vi "Text control 2 v0.8.vi"() -> ()   [LabVIEW 2016]
panel:
  out "error out":errorcluster
  in  "Units":bool
  out "Elapsed Time":dbl caption="Elapsed Time (s)"
  out "Ion vs time":cluster{"Y data in":dbl[], "X data in":dbl[]}[](graph)
  out "Ig":dbl format="%.2e"
  out "Id":dbl format="%.2e"
  out "Is":dbl format="%.2e"
  out "I vs Vg":cluster{"Y data in":dbl[], "X data in":dbl[]}[](graph)
  in  "Panel Controls 2":T1={"Emergency Stop"=refnum, "TransGraph Max"=1e-05, "Text/Graph (text=false)"=TRUE, "TransGraph Min"=1e-11} {"TransGraph Min" format="%.2e"; "TransGraph Max" format="%.2e"}
  out "Currently running:":string="#output s 0 0 0 -0.008 0.008 0.002"
  in  "Lines left to run:":string
  in  "Standby":T2
  in  "Full Reset":bool
  in  "SMU4":cluster{"on/off":bool, "Voltage":dbl} {"Voltage" min=-100.0 max=100.0 format="%.2f"}
  in  "Source/Drain Range":u8(slide)=6 max=11 scale=0.0..11.0
  in  "Source/Drain\nRange mode":u16(ring) items=["Auto", "Limited", "Fixed"]
  in  "Gate Range":u8(slide)=6 max=11 scale=0.0..11.0
  in  "Gate Range\nmode":u16(ring) items=["Auto", "Limited", "Fixed"]
  in  "Gate":T3={"Gate Start"=0.0, "Gate Stop"=2.0, "Gate Step (linear only)"=1.0, "Gate Compliance"=0.0001, "Gate PComp"=0.0, "Range mode"=0, "Range"=6} {"Range" max=11 scale=0.0..11.0; "Range mode" items=["Auto", "Limited", "Fixed"]; "Gate PComp" format="%^.2e"; "Gate Compliance" format="%^.2e"; "Gate Step (linear only)" format="%^.4e"; "Gate Stop" format="%^.4e"; "Gate Start" format="%^.4e"}
  in  "Drain 2":T4={"Drain Start"=0.0, "Drain Stop"=2.0, "Drain Compliance"=0.0001, "Drain Step"=1.0, "Drain PComp"=0.0, "Range mode"=0, "Range"=6} {"Range" max=11 scale=0.0..11.0; "Range mode" items=["Auto", "Limited", "Fixed"]; "Drain PComp" format="%^.2e"; "Drain Step" format="%^.4e"; "Drain Compliance" format="%^.2e"; "Drain Stop" format="%^.4e"; "Drain Start" format="%^.4e"}
  in  "Timings 2":T5={"integration time"=0, "Short/Long integration time"=0.00064, "hold time (sec)"=0.0, "delay time (sec)"=0.0, "Step Time (0 disables)"=0.0, "sweep method"=0, "Pulse period"=0.005, "Base voltage"=0.0, "Pulse width"=0.0005} {"Pulse width" min=0.0005 max=0.1 step=0.0001 format="%.4f"; "Base voltage" format="%^.4e"; "Pulse period" min=0.005 max=1.0 step=0.0001 format="%.4f"; "sweep method" items=["Continuous", "Pulsed"]; "Step Time (0 disables)" format="%.2f"; "delay time (sec)" format="%.4f"; "hold time (sec)" format="%.4f"; "Short/Long integration time" format="%^.0e"; "integration time" scale=0.0..2.0}
  in  "Panel Controls":T6={"Emergency Stop"=refnum, "TransGraph Max"=1e-05, "Text/Graph (text=false)"=TRUE} {"TransGraph Max" format="%.2e"}
  in  "Interrupt run":bool
  in  "Drain: Compliance":dbl=0.001 format="%.8f"
  in  "Gate: Compliance":dbl=0.001 format="%.8f"
  out "Path":path=path "C:/users/rlp38/09Apr2009LTtesting/test2.txt"
  in  "hold time /s":dbl format="%.2f"
  in  "delay time /s":dbl format="%.2f"
  in  "integration time":u32(slide) max=2 step=1 scale=0.0..2.0
  in  "Integration time (short)":dbl=0.0019 min=8e-05 max=0.0019 step=8e-05 format="%^.0e"
  in  "Integration time (long)":dbl=0.32 min=0.04 max=2.0 step=0.02 format="%.2f"
  in  "Step delay /s":dbl format="%.2f"
  in  "Program":string="#pulsedstressV d 0.03 20 0 0.5 0.0827 5\n#\nitime s\ngaterangemode l\ndrainrangemode l\n#pulsed on 0.05 0 0.02\ntransfer d 1 -1 -0.1 -1 -1 0\nwait-min 1\ntransfer d 1 -1 -0.1 -1 -1 0\n#transfer d -10 40 1 5 40 35\n#transfer d -10 40 1 5 40 35\n#output d 0 40 20 0 40 1\n#\n#\n#sample 1 0.008 221 6 0.003\n#samplei 400e-6 200 6 0.002 0.1\n#vsu2pulse -10 4\n#\n#stressV 0.016 0.03 2e-4 0.1e-3 11\n#stressI 220e-7 0.08 15\n#transfer s -1 1 0.5 -0.005 0.005 0.005\n#output s 0 0 0 -0.008 0.008 0.002\n"
  # "Syntax:\nitime [s|m|l]\ngaterangemode [a|l|f]\ndrainrangemode [a|l|f]\npulsed [on|off] PulsePeriod(sec) PulseBaseVoltage PulseONWidth(sec)\nstandby [on l off]\nwait NumMilliseconds\nwait-min NumMinutes\n# texthere = comment\ntransfer [s|d] VgStart VgStop VgStep VdStart VdStop VdStep\noutput [s|d] VgStart VgStop VgStep VdStart VdStop VdStep\nsample Vg Vd NumSamples Time(s) SampleInterval(s)\nsamplei Idg NumSamples Time(s) SampleInterval(s) VDGcompliance\n# if in doubt use SampleInterval(s) = 0.004\nstressV VG VD IGcompliance IDcompliance Duration(sec)\nstressI IDG VDGcompliance Duration(sec)\nvsu2pulse Bias Duration(s)\npulsedstressV [s|d] VEstop VgON VgOFF Period(s) PulseONwidth(s) Vd\nsample-fpp Vg Vd NumSamples Time\nresample-fpp Vg Vd\ntransfer-fpp [s|d] VgStart VgStop VgStep VdStart VdStop VdStep\noutput-fpp [s|d] VgStart VgStop VgStep VdStart VdStop VdStep"
  # "Time"
  # "Sec"
  # "Min"
  # "100 samples is approx 13s with medium integration"
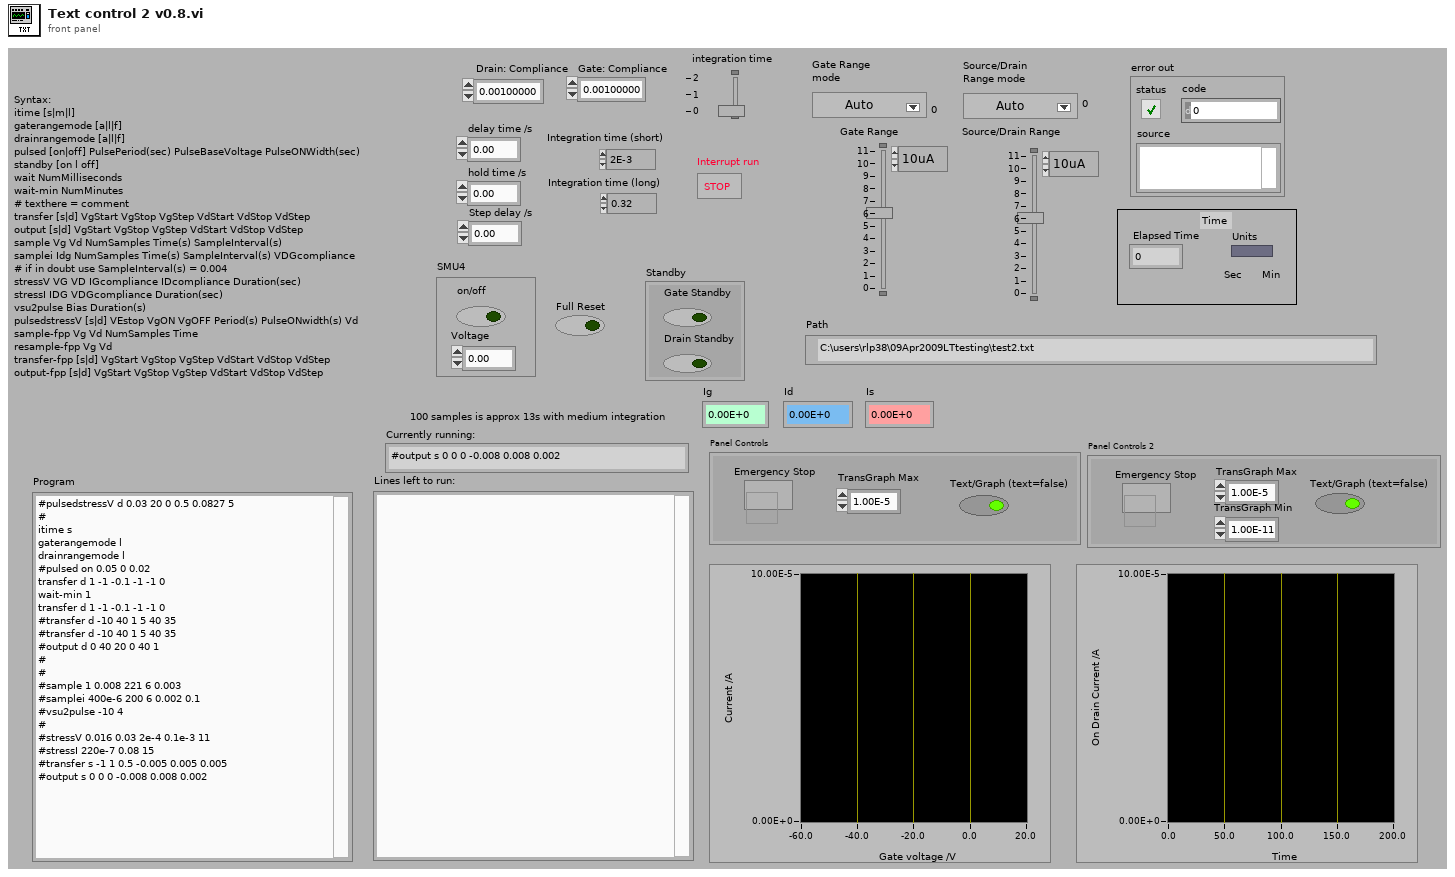
[diagram p1: front panel]
types:
  T1 = cluster{"Emergency Stop":refnum<vi>, "TransGraph Max":dbl, "Text/Graph (text=false)":bool, "TransGraph Min":dbl}
  T2 = cluster{"Gate Standby":bool, "Drain Standby":bool}
  T3 = cluster{"Gate Start":dbl, "Gate Stop":dbl, "Gate Step (linear only)":dbl, "Gate Compliance":dbl, "Gate PComp":dbl, "Range mode":u16, "Range":u8}
  T4 = cluster{"Drain Start":dbl, "Drain Stop":dbl, "Drain Compliance":dbl, "Drain Step":dbl, "Drain PComp":dbl, "Range mode":u16, "Range":u8}
  T5 = cluster{"integration time":u32, "Short/Long integration time":dbl, "hold time (sec)":dbl, "delay time (sec)":dbl, "Step Time (0 disables)":dbl, "sweep method":u16, "Pulse period":dbl, "Base voltage":dbl, "Pulse width":dbl}
  T6 = cluster{"Emergency Stop":refnum<vi>, "TransGraph Max":dbl, "Text/Graph (text=false)":bool}
  T7 = enum16{"open", "replace", "create", "open or create", "replace or create", "replace or create with confirmation"}
  T8 = cluster{"V2 Start":dbl, "V2 Step":dbl, "Number of points":i32}
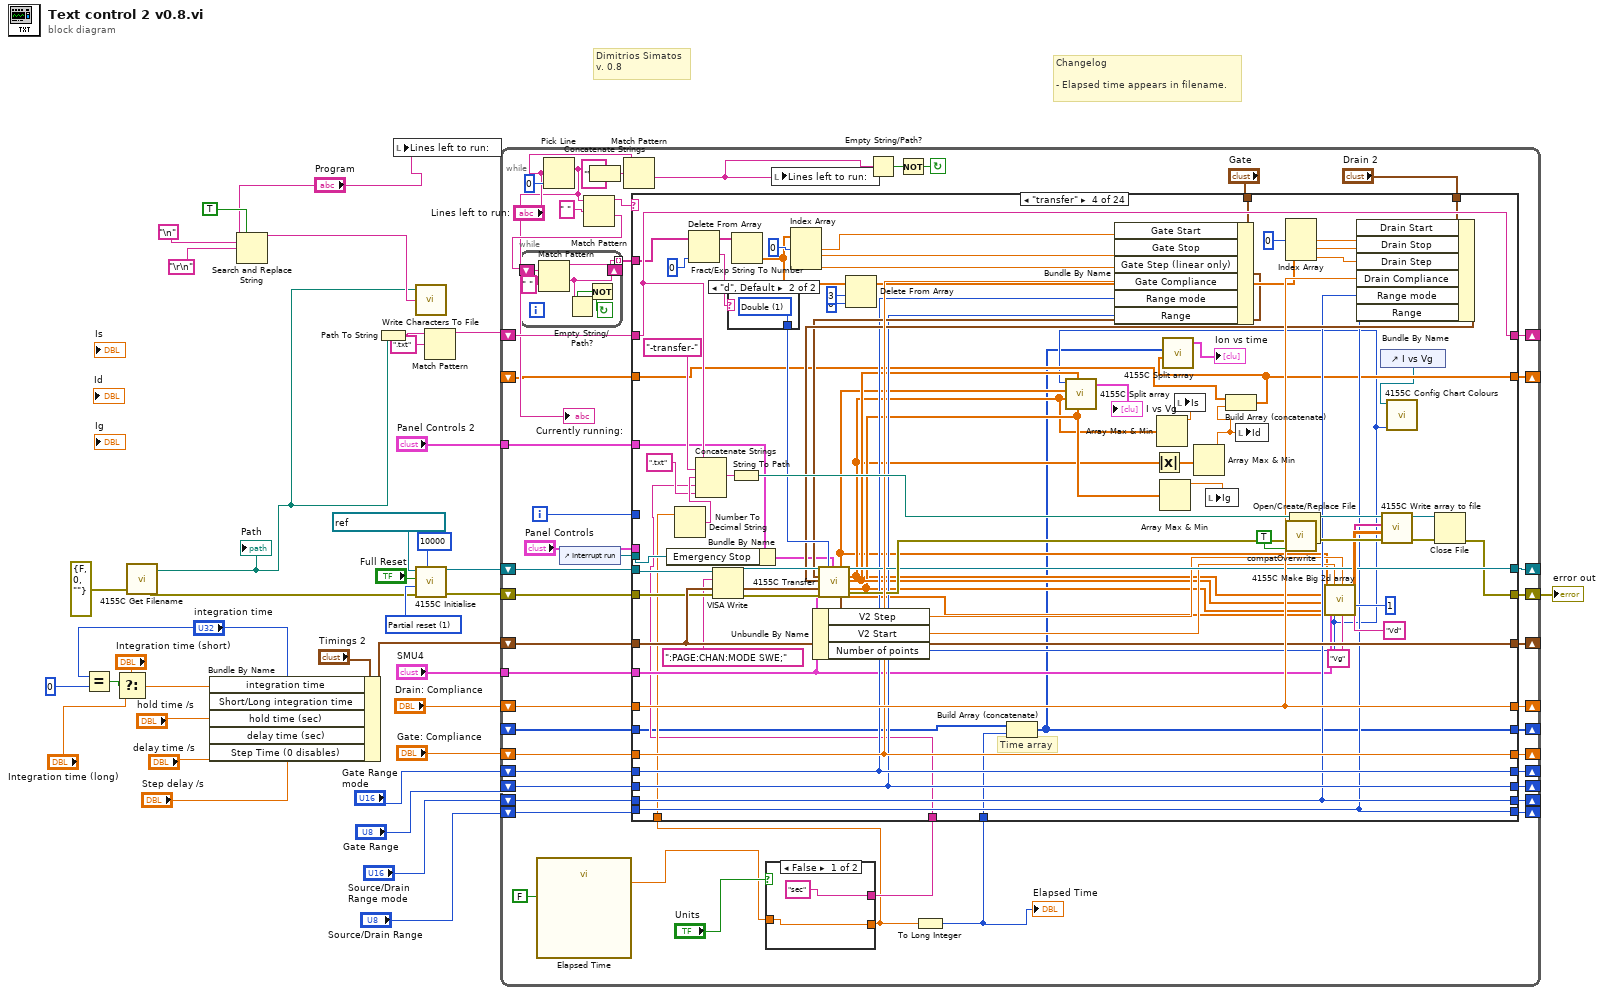
[diagram p0: block diagram]
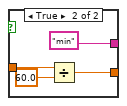
[diagram p2: hidden frame]
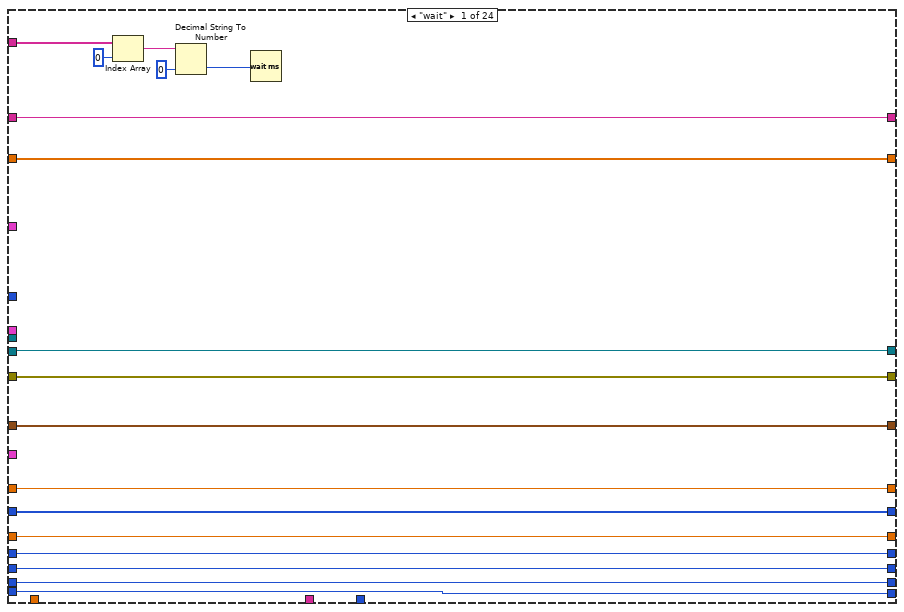
[diagram p3: hidden frame]
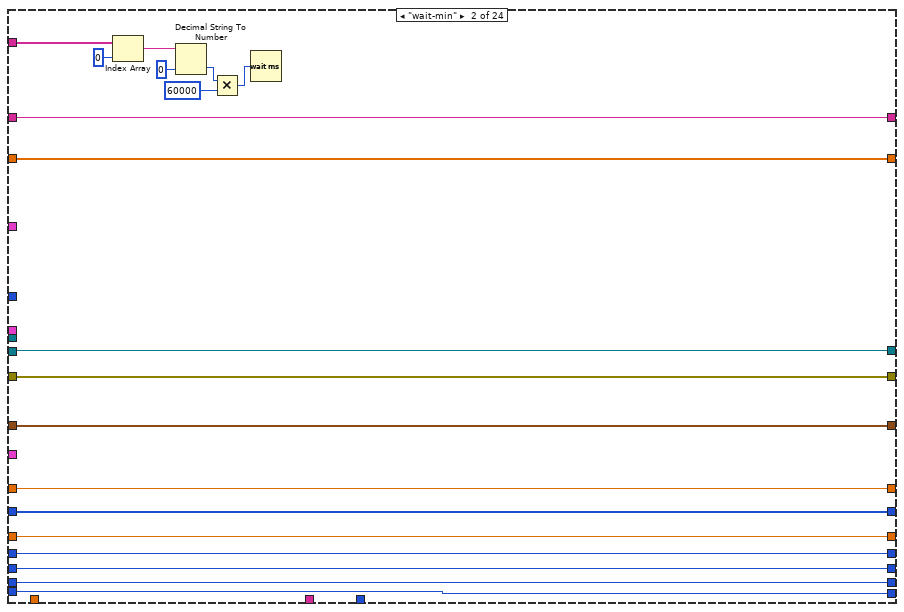
[diagram p4: hidden frame]
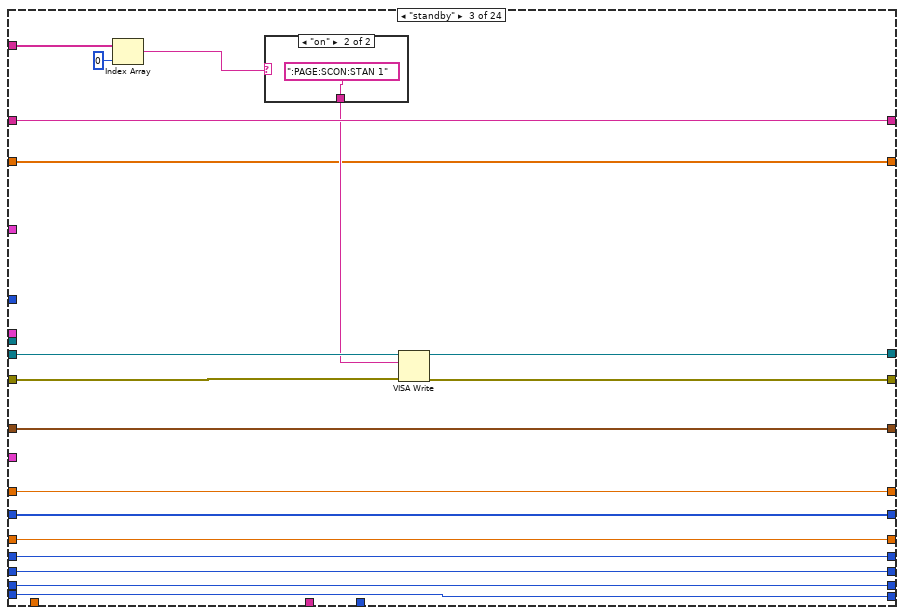
[diagram p5: hidden frame]
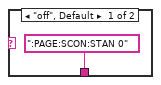
[diagram p6: hidden frame]
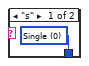
[diagram p7: hidden frame]
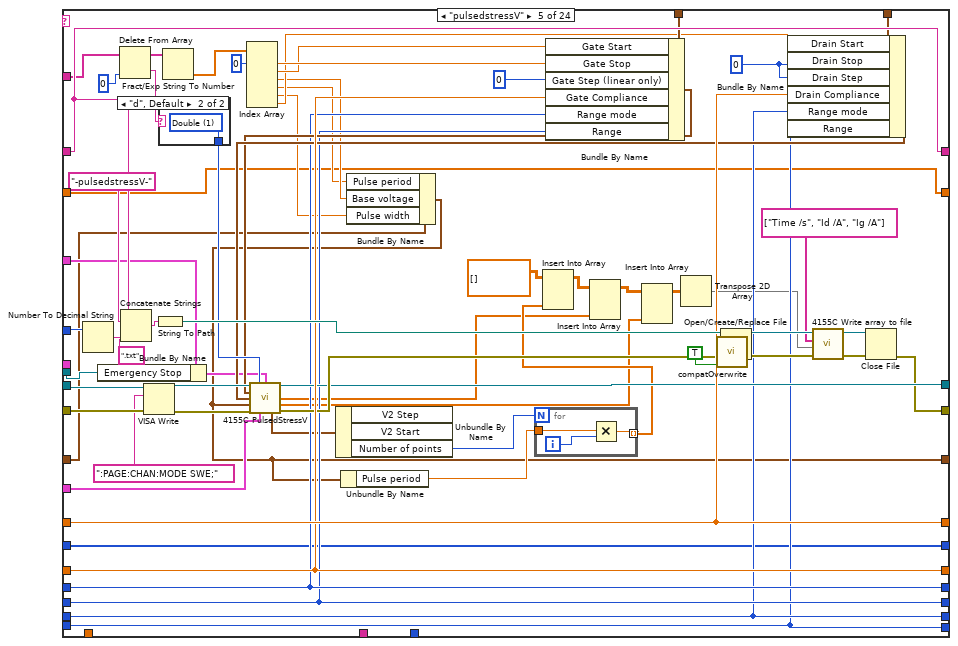
[diagram p8: hidden frame]
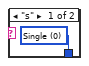
[diagram p9: hidden frame]
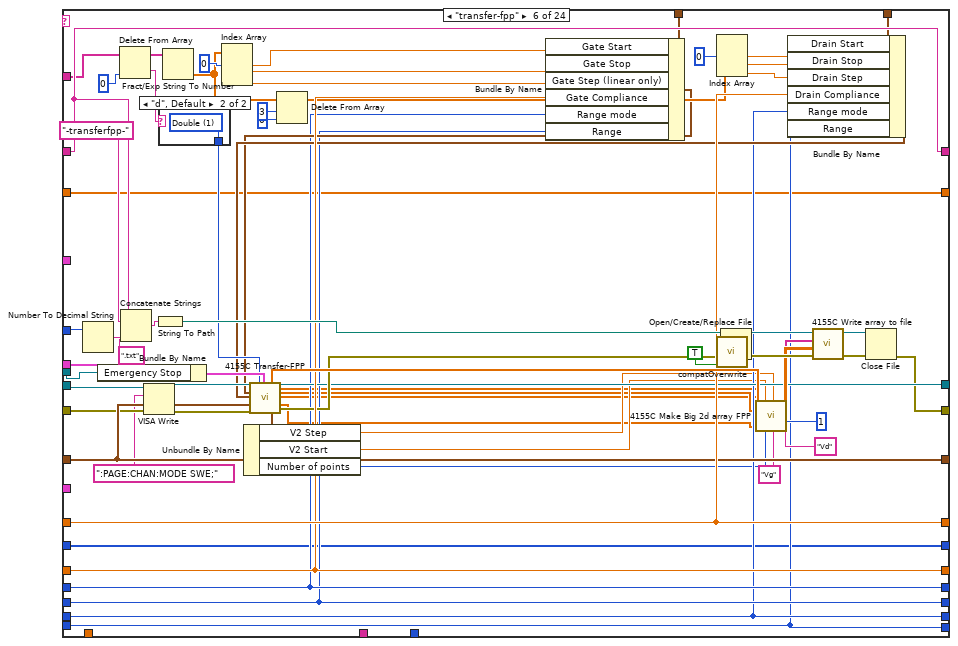
[diagram p10: hidden frame]
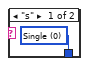
[diagram p11: hidden frame]
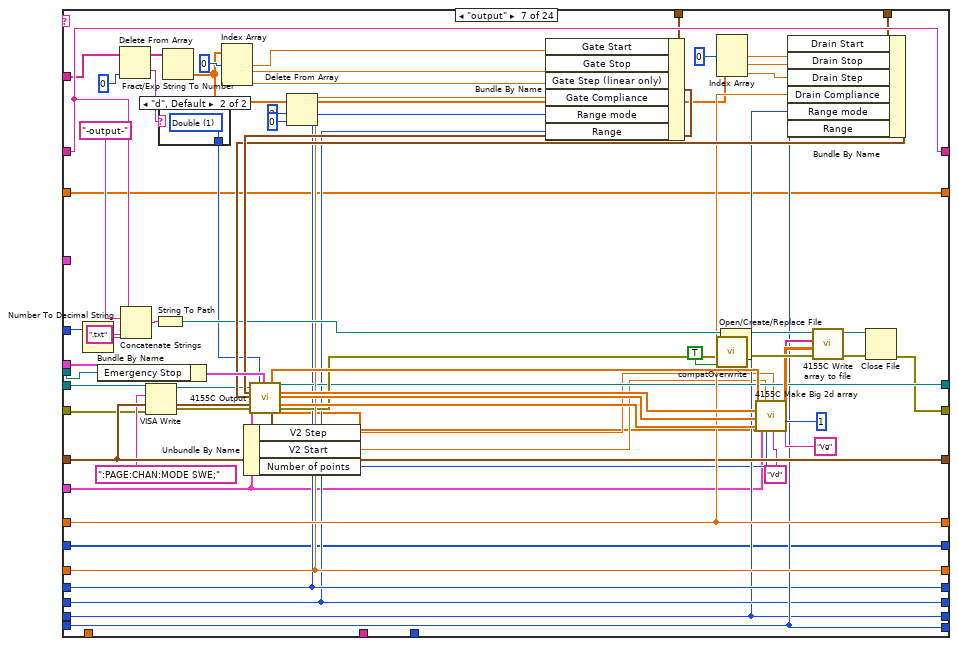
[diagram p12: hidden frame]
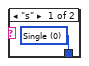
[diagram p13: hidden frame]
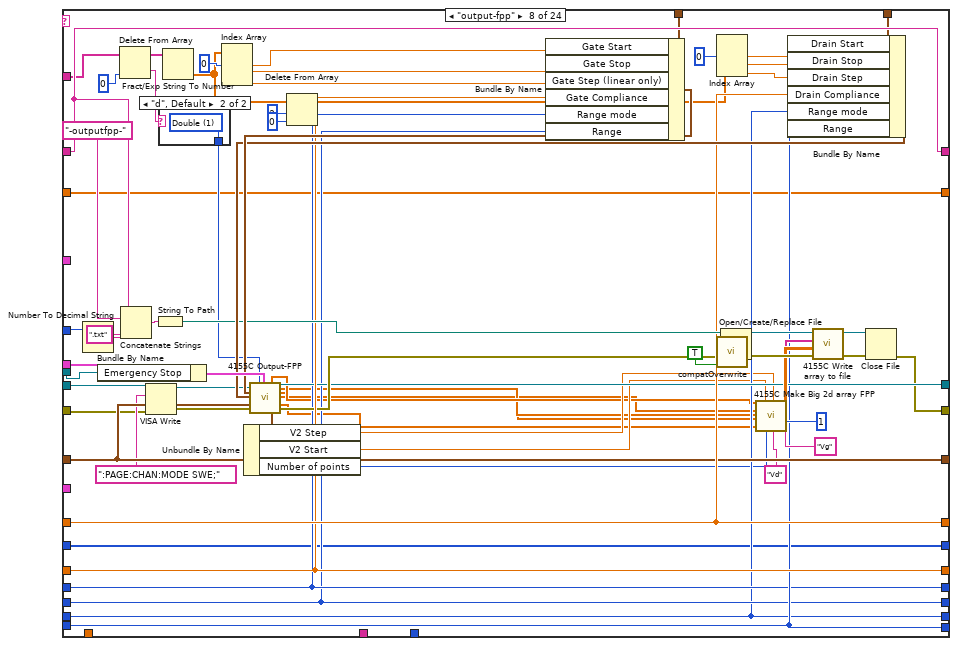
[diagram p14: hidden frame]
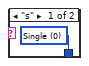
[diagram p15: hidden frame]
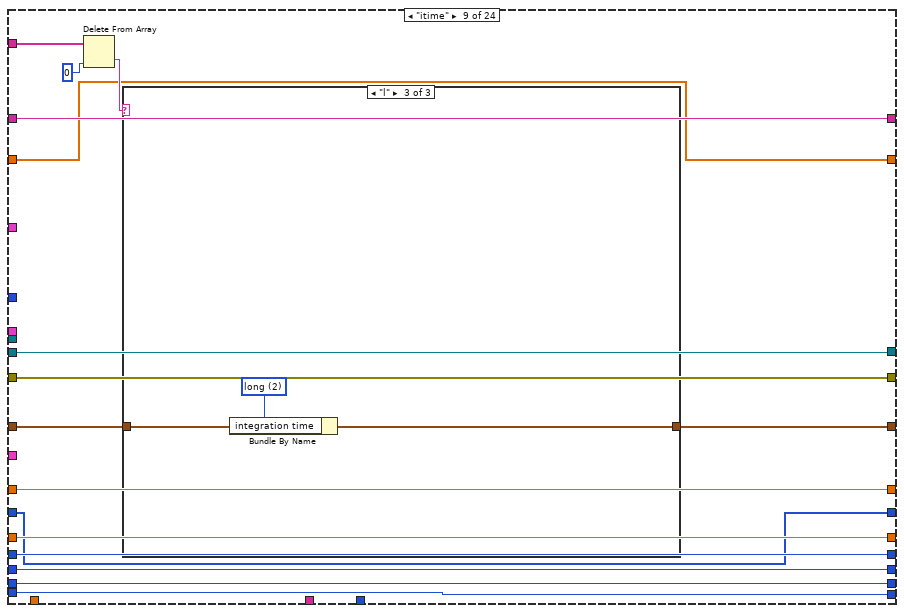
[diagram p16: hidden frame]
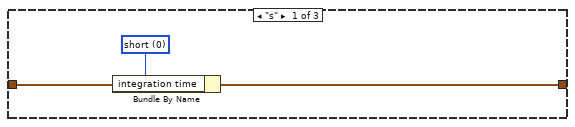
[diagram p17: hidden frame]
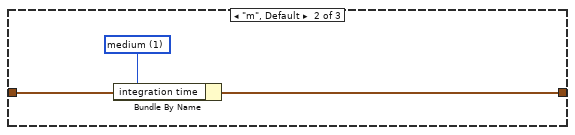
[diagram p18: hidden frame]
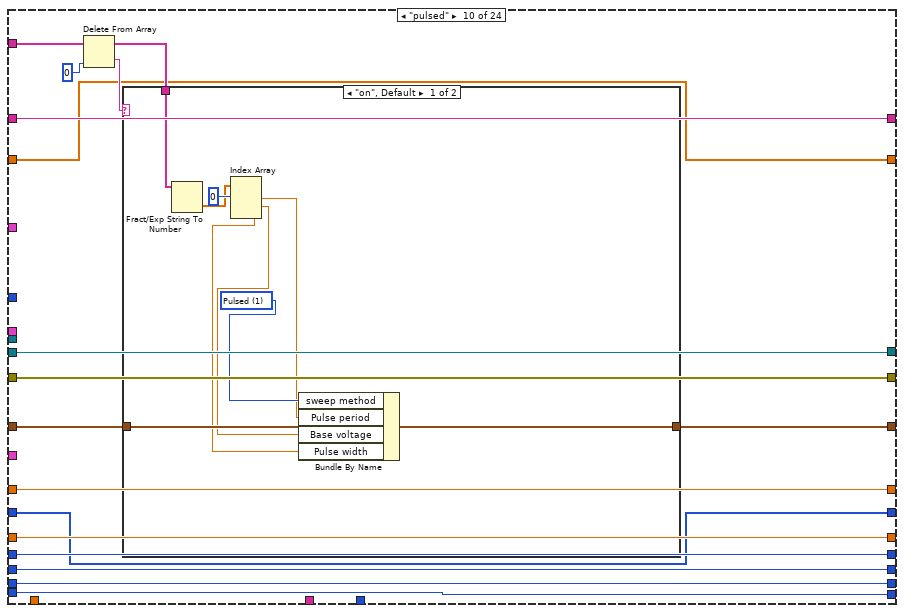
[diagram p19: hidden frame]
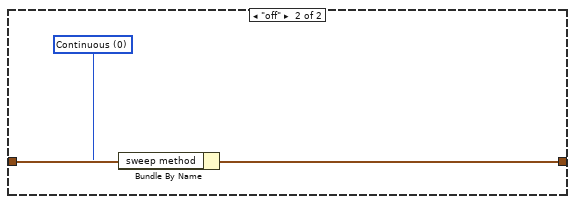
[diagram p20: hidden frame]
diagram:
  w28 = u16 1 items=["Reset All", "Partial reset"] ("Type of reset")
  # "Dimitrios Simatos\nv. 0.8"
  # "Changelog\n\n- Elapsed time appears in filename."
  n1 = Equal?(x="integration time", y=u32 0) -> (x = y?=w32:bool)
  n2 = Select(t="Integration time (short)", s=w32, f="Integration time (long)") -> (s? t:f=w36:dbl)
  n3 = call <userlib>:"4155C Get Filename.vi"("error in (no error)"=errorcluster {"status"=FALSE, "code"=0, "source"=""}) -> ("error out"=w23:errorcluster, "path"=w7:path)  [unwired: 2 in, 1 out]
  "Path" <- w7
  n4 = Bundle By Name(cluster="Timings 2", "integration time"="integration time", "Short/Long integration time"=w36, "hold time (sec)"="hold time /s", "delay time (sec)"="delay time /s", "Step Time (0 disables)"="Step delay /s") -> (w20:T5)
  n5 = Search and Replace String(replace all?=TRUE ("replace all? (F)"), input string="Program", search string="\n", replace string="\r\n") -> (result string=w10:string)  [unwired: 4 in, 3 out]
  n6 = Path To String(path=w7) -> (string=w6:string)
  n7 = local write "Lines left to run:"("Program") -> ()
  n8 = call <vilib>:"Write Characters To File.vi"("character string"=w10, "file path (dialog if empty)"=w7) -> ()  [unwired: 3 in, 1 out]
  n9 = call <userlib>:"4155C Initialise.vi"("VISA resource name in"=refnum<visa-resource-name> "GPIB0::14::INSTR", "Reset"="Full Reset", "Type of reset"=w28, "error in (no error)"=w23, "VISA Timeout Value"=u32 10000) -> ("VISA Resource Name out"=w22:refnum<visa-resource-name>, "error out"=w21:errorcluster)
  n10 = Match Pattern(string=w6, regular expression=".txt") -> (before substring=w5:string)  [unwired: 1 in, 3 out]
  n11 = while {
    tunnel: "SMU4" -> [w52]
    shift-left: "Source/Drain Range" -> [w57]
    shift-right: [w53] -> _
    shift-left: "Source/Drain\nRange mode" -> [w58]
    shift-right: [w54] -> _
    shift-left: "Gate Range" -> [w59]
    shift-right: [w55] -> _
    shift-left: "Gate Range\nmode" -> [w60]
    shift-right: [w56] -> _
    shift-left: "Gate: Compliance" -> [w72]
    shift-right: [w66] -> _
    shift-left: "Drain: Compliance" -> [w73]
    shift-right: [w67] -> _
    shift-left: w20 -> [w74]
    shift-right: [w68] -> _
    shift-left: w21 -> [w75]
    shift-right: [w69] -> w1
    shift-left: w22 -> [w76]
    shift-right: [w70] -> _
    shift-left: w5 -> [w77]
    shift-right: [w65] -> _
    tunnel: "Panel Controls 2" -> [w48]
    shift-right: [w47] -> _
    shift-left: _ -> [w46]
    shift-right: [w41] -> _
    shift-left: _ -> [w40]
    i -> [w71]
    stop <- w85 continue-if-true
    n12 = call "Elapsed Time"("Auto Reset"=FALSE) -> ("Elapsed Time (s)"=w42:dbl)  [unwired: 11 in, 7 out]
    n13 = Pick Line(multi-line string="Lines left to run:", line index=0) -> (output string=w49:string)  [unwired: 1 in]
    "Currently running:" <- w49
    n14 = control-ref of="Interrupt run"() -> (w64:refnum<vi>)
    n15 = Match Pattern(string=w49, regular expression=" ") -> (before substring=w80:string, after substring=w79:string)  [unwired: 1 in, 2 out]
    n16 = while {
      tunnel: [w93] -> w78 mode=indexing
      shift-left: w79 -> [w95]
      shift-right: [w94] -> _
      stop <- w97 continue-if-true
      n17 = Match Pattern(string=w95, regular expression=" ") -> (before substring=w93:string, after substring=w94:string)  [unwired: 1 in, 2 out]
      n18 = Empty String/Path?(string/path=w94) -> (empty?=w98:bool)
      n19 = Not(x=w98) -> (.not. x?=w97:bool)
    }
    n20 = Concatenate Strings(w49, "\n" ("Substring")) -> (w83:string)
    n21 = Match Pattern(string="Lines left to run:", regular expression=w83) -> (after substring=w50:string)  [unwired: 1 in, 3 out]
    n22 = case shown="False" "Units" {
      tunnel: ["sec" "min"] -> w43
      tunnel: [w87 w91] -> w39
      tunnel: w42 -> [w87 w90]
      frame False {
      }
      frame True {
        n23 = Divide(x=w90, y=60.0) -> (x/y=w91:dbl)
      }
    }
    n24 = local write "Lines left to run:"(w50) -> ()
    n25 = Empty String/Path?(string/path=w50) -> (empty?=w86:bool)
    n26 = Not(x=w86) -> (.not. x?=w85:bool)
    n27 = To Long Integer(number=w39) -> (32bit integer=w38:i32)
    "Elapsed Time" <- w38
    n28 = case shown="\"transfer\"" w80 {
      tunnel: w78 -> [w115 w134 w152 w216 w285 w353 w419 w493 w532 w558 w585 w610 w631 w645 _ _ w746 w806 _ w870 w913 w954 w1023 w1084]
      tunnel: w77 -> [w110 w130 w150 w224 w292 w361 w427 w501 w521 w547 w577 w603 w625 w638 w657 w697 w724 w788 w820 w857 w900 w942 w1017 w1080]
      tunnel: w76 -> [w109 w129 w141 w194 w276 w330 w395 w469 w522 w548 w578 w604 w626 w639 w662 w700 w753 w813 w824 w877 w920 w961 w1030 w1037]
      tunnel: w75 -> [w108 w128 w140 w193 w275 w329 w392 w466 w523 w549 w579 w605 w627 w640 w661 w669 w752 w812 w823 w876 w919 w960 w1029 w1036]
      tunnel: w74 -> [w107 w127 w149 w220 w250 w357 w423 w497 w531 w557 w576 w602 w624 w637 w660 w693 w715 w780 w829 w850 w893 w935 w1016 w1079]
      tunnel: w73 -> [w106 w126 w148 w222 w290 w359 w425 w499 w530 w556 w584 w609 w630 w644 w659 w678 w751 w811 w832 w875 w918 w959 w1028 w1089]
      tunnel: w72 -> [w105 w125 w147 w221 w289 w358 w424 w498 w529 w555 w583 w608 w629 w643 w658 w679 w725 w789 w831 w858 w901 w943 w1018 w1081]
      tunnel: w71 -> [_ _ _ _ w293 w362 w428 w502 _ _ _ _ _ _ _ w695 w750 w810 _ w874 w917 w958 w1027 w1088]
      tunnel: [w109 w129 w139 w218 w287 w355 w421 w495 w522 w548 w578 w604 w626 w639 w662 w700 w716 w761 w822 w851 w894 w936 w968 w1039] -> w70
      tunnel: [w108 w128 w138 w217 w286 w354 w420 w494 w523 w549 w579 w605 w627 w640 w661 w668 w726 w762 w821 w859 w902 w944 w967 w1038] -> w69
      tunnel: [w107 w127 w149 w220 w246 w357 w423 w497 w524 w550 w576 w602 w624 w637 w660 w693 w715 w780 w829 w850 w893 w935 w1016 w1079] -> w68
      tunnel: [w106 w126 w148 w222 w290 w359 w425 w499 w530 w556 w584 w609 w630 w644 w659 w678 w751 w811 w832 w875 w918 w959 w1028 w1089] -> w67
      tunnel: [w105 w125 w147 w221 w289 w358 w424 w498 w529 w555 w583 w608 w629 w643 w658 w679 w725 w789 w831 w858 w901 w943 w1018 w1081] -> w66
      tunnel: [w110 w130 w150 w224 w292 w361 w427 w501 w521 w547 w577 w603 w625 w638 w657 w697 w724 w788 w820 w857 w900 w942 w1017 w1080] -> w65
      tunnel: w64 -> [_ _ _ w227 w297 w367 w436 w506 _ _ _ _ _ _ _ _ w721 w785 _ w856 w899 w941 w988 w1055]
      tunnel: "Gate" -> [_ _ _ w203 w279 w340 w406 w480 _ _ _ _ _ _ _ _ _ _ _ _ _ _ _ _]
      tunnel: "Drain 2" -> [_ _ _ w202 w278 w339 w405 w479 _ _ _ _ _ _ _ _ _ _ _ _ _ _ _ _]
      tunnel: "Panel Controls" -> [_ _ _ _ _ w338 w404 w478 _ _ _ _ _ _ _ _ _ _ _ _ _ _ _ _]
      tunnel: w60 -> [w104 w124 w146 w187 w269 w323 w390 w464 w528 w554 _ w601 w623 w636 w656 w680 w711 w776 w825 w846 w889 w931 w1012 w1075]
      tunnel: w59 -> [w103 w123 w145 w186 w268 w322 w389 w463 w527 w553 w582 _ w614 w642 w655 w681 w712 w777 w826 w847 w890 w932 w1013 w1076]
      tunnel: w58 -> [w102 w122 w144 w185 w267 w321 w388 w462 w526 w552 w581 w607 w628 _ w654 w682 w713 w778 w827 w848 w891 w933 w1014 w1077]
      tunnel: w57 -> [w101 w121 w143 w184 w266 w320 w391 w465 w525 w551 w580 w606 _ w641 w653 w683 w714 w779 w828 w849 w892 w934 w1015 w1078]
      tunnel: [w104 w124 w146 w187 w269 w323 w390 w464 w528 w554 w575 w601 w623 w636 w656 w680 w711 w776 w825 w846 w889 w931 w1012 w1075] -> w56
      tunnel: [w103 w123 w145 w186 w268 w322 w389 w463 w527 w553 w582 w593 w614 w642 w655 w681 w712 w777 w826 w847 w890 w932 w1013 w1076] -> w55
      tunnel: [w102 w122 w144 w185 w267 w321 w388 w462 w526 w552 w581 w607 w628 w635 w654 w682 w713 w778 w827 w848 w891 w933 w1014 w1077] -> w54
      tunnel: [w101 w121 w143 w184 w266 w320 w391 w465 w525 w551 w580 w606 w615 w641 w653 w683 w714 w779 w828 w849 w892 w934 w1015 w1078] -> w53
      tunnel: w52 -> [_ _ _ w179 w262 _ w382 _ _ _ _ _ _ _ _ _ _ _ _ _ _ _ _ _]
      tunnel: w48 -> [_ _ _ w177 w261 _ _ _ _ _ _ _ _ _ _ _ _ _ _ _ _ _ _ _]
      tunnel: [w100 w117 w136 w166 w238 w309 w379 w450 w520 w545 w574 w592 w613 w634 w652 w664 w702 w759 w819 w834 w881 w924 w965 w1032] -> w47
      tunnel: w46 -> [w100 w117 w136 w165 w238 w309 w379 w450 w520 w545 w574 w592 w613 w634 w652 w664 w702 w759 w819 w834 w881 w924 w965 w1032]
      tunnel: w39 -> [_ _ _ w161 _ _ _ _ _ _ _ _ _ _ _ _ _ _ _ _ _ _ _ _]
      tunnel: w43 -> [_ _ _ w158 _ _ _ _ _ _ _ _ _ _ _ _ _ _ _ _ _ _ _ _]
      tunnel: w38 -> [_ _ _ w155 _ _ _ _ _ _ _ _ _ _ _ _ _ _ _ _ _ _ _ _]
      tunnel: [w99 w116 w135 w157 w237 w308 w378 w449 w519 w544 w573 w591 w612 w633 w651 w663 w701 w758 w818 w833 w880 w923 w964 w1031] -> w41
      tunnel: w40 -> [w99 w116 w135 w156 w237 w308 w378 w449 w519 w544 w573 w591 w612 w633 w651 w663 w701 w758 w818 w833 w880 w923 w964 w1031]
      frame "wait" {
        n29 = Index Array(array=w115, index=0 ("Index")) -> (element=w113:string)
        n30 = Decimal String To Number(string=w113, default (0L)=u32 0) -> (number=w112:u32)  [unwired: 1 in, 1 out]
        n31 = Wait (ms)(milliseconds to wait=w112) -> ()  [unwired: 1 out]
      }
      frame "wait-min" {
        n32 = Index Array(array=w134, index=0 ("Index")) -> (element=w132:string)
        n33 = Decimal String To Number(string=w132, default (0L)=u32 0) -> (number=w120:u32)  [unwired: 1 in, 1 out]
        n34 = Multiply(x=w120, y=u32 60000) -> (x*y=w119:u32)
        n35 = Wait (ms)(milliseconds to wait=w119) -> ()  [unwired: 1 out]
      }
      frame "standby" {
        n36 = Index Array(array=w152, index=0 ("Index")) -> (element=w142:string)
        n37 = case shown="\"on\"" w142 {
          tunnel: [":PAGE:SCON:STAN 0" ":PAGE:SCON:STAN 1"] -> w137
          frame "off", Default {
          }
          frame "on" {
          }
        }
        n38 = VISA Write(VISA resource name=w141, write buffer=w137, error in (no error)=w140) -> (VISA resource name out=w139:refnum<visa-resource-name>, error out=w138:errorcluster)  [unwired: 1 out]
      }
      frame "transfer" {
        # "Time array"
        n39 = Bundle By Name(cluster=w177, "Emergency Stop"=w227) -> (w178:T1)
        n40 = Number To Decimal String(number=w161) -> (decimal integer string=w160:string)  [unwired: 1 in]
        n41 = Delete From Array(array=w216, index=0 ("Index")) -> (deleted portion=w214:string, array with subset deleted=w213:string[])  [unwired: 1 in]
        n42 = Concatenate Strings(w224, "-transfer-" ("Prefix"), w160, w158, ".txt" ("Suffix")) -> (w226:string)
        n43 = VISA Write(VISA resource name=w194, write buffer=":PAGE:CHAN:MODE SWE;" ("write buffer (\"\")"), error in (no error)=w193) -> (VISA resource name out=w191:refnum<visa-resource-name>, error out=w192:errorcluster)  [unwired: 1 out]
        n44 = case shown="\"d\", Default" w214 {
          tunnel: [w235 w236] -> w212
          frame "s" {
            w235 = u16 0 items=["Single", "Double"] ("sweep mode")
          }
          frame "d", Default {
            w236 = u16 1 items=["Single", "Double"] ("sweep mode")
          }
        }
        n45 = String To Path(string=w226) -> (path=w223:path)
        n46 = Fract/Exp String To Number(string=w213) -> (number=w198:dbl[])  [unwired: 3 in, 1 out]
        n47 = Index Array(array=w198, index #1=0 ("Index")) -> (element #1=w211:dbl, element #2=w210:dbl, element #3=w209:dbl)  [unwired: 2 in]
        n48 = Delete From Array(array=w198, length=3 ("Length"), index=0 ("Index")) -> (array with subset deleted=w196:dbl[])  [unwired: 1 out]
        n49 = Build Array (concatenate)(w156, w155) -> (w157:i32[])
        n50 = Bundle By Name(cluster=w203, "Gate Start"=w211, "Gate Stop"=w210, "Gate Step (linear only)"=w209, "Gate Compliance"=w221, "Range mode"=w187, "Range"=w186) -> (w188:T3)
        n51 = Index Array(array=w196, index #1=0 ("Index")) -> (element #1=w206:dbl, element #2=w205:dbl, element #3=w204:dbl)  [unwired: 2 in]
        n52 = call <vilib>:"compatOverwrite.vi"("overwrite (F)"=TRUE) -> ("overwrite?"=w176:T7)
        n53 = Bundle By Name(cluster=w202, "Drain Start"=w206, "Drain Stop"=w205, "Drain Step"=w204, "Drain Compliance"=w222, "Range mode"=w185, "Range"=w184) -> (w189:T4)
        n54 = call <userlib>:"4155C Transfer.vi"("VISA resource name in"=w191, "Gate"=w188, "Drain"=w189, "Timings"=w220, "error in (no error)"=w192, "SMU4"=w179, "sweep mode"=w212, "Panel Controls"=w178) -> ("VG"=w167:dbl[], "Outparams"=w183:T8, "VISA Resource Name out"=w218:refnum<visa-resource-name>, "IS"=w169:dbl[], "ID"=w174:dbl[], "IG"=w170:dbl[], "error out"=w219:errorcluster, "SMU4"=w180:dbl[])  [unwired: 12 in]
        n55 = Unbundle By Name(w183) -> ("V2 Step"=w182:dbl, "V2 Start"=w181:dbl, "Number of points"=w163:i32)
        n56 = call <userlib>:"4155C Split array.vi"("Number of VAR2 steps"=w163, "Y2 data in"=w174, "X data in"=w167, "Y1 data in"=w169, "Y3 data in"=w170) -> ("Array of clusters"=→"I vs Vg":cluster{"Y data in":dbl[], "X data in":dbl[]}[])  [unwired: 2 in, 1 out]
        n57 = Absolute Value(x=w169) -> (abs(x)=w173:dbl[])
        n58 = Array Max & Min(array=w169) -> (max value=w171:dbl)  [unwired: 3 out]
        n59 = Array Max & Min(array=w170) -> (max value=w172:dbl)  [unwired: 3 out]
        n60 = local write "Is"(w171) -> ()
        n61 = Array Max & Min(array=w173) -> (max value=w164:dbl)  [unwired: 3 out]
        n62 = local write "Ig"(w172) -> ()
        n63 = Build Array (concatenate)(w165, w164) -> (w166:dbl[])
        n64 = call <userlib>:"4155C Split array.vi"("X data in"=w157, "Y1 data in"=w166) -> ("Array of clusters"=→"Ion vs time":cluster{"Y data in":dbl[], "X data in":dbl[]}[])  [unwired: 5 in, 1 out]
        n65 = local write "Id"(w164) -> ()
        n66 = Open/Create/Replace File(file path (use dialog)=w223, error in=w219, operation (0:open)=w176) -> (refnum out=w232:refnum<file>, error out=w233:errorcluster)  [unwired: 3 in, 1 out]
        n67 = call <userlib>:"4155C Make Big 2d array.vi"("1D Var1"=w167, "1d IS"=w169, "1d ID"=w174, "1d IG"=w170, "1d SMU4"=w180, "SMU4"=w179, "VAR2 START"=w181, "Number of VAR2 steps"=w163, "VAR2 STEP"=w182, "VAR1 Name"="Vg", "Decimal places in header"=i8 1, "VAR2 Name"="Vd") -> ("Header array"=w228:string[], "Data array"=w229:dbl[][])  [unwired: 14 in]
        n68 = control-ref of="I vs Vg"() -> (w162:refnum<vi>)
        n69 = call <userlib>:"4155C Write array to file.vi"("Byte Stream File Refnum"=w232, "Header"=w228, "Data Array"=w229, "error in (no error)"=w233) -> ("dup refnum"=w230:refnum<file>, "error out"=w231:errorcluster)  [unwired: 1 in]
        n70 = call <userlib>:"4155C Config Chart Colours.vi"("Numeric"=w163, "XY Graph 2"=w162) -> ()  [unwired: 6 in]
        n71 = Close File(refnum=w230, error in=w231) -> (error out=w217:errorcluster)  [unwired: 1 out]
      }
      frame "pulsedstressV" {
        w244 = 0
        n72 = Number To Decimal String(number=w293) -> (decimal integer string=w294:string)  [unwired: 1 in]
        n73 = Bundle By Name(cluster=w261, "Emergency Stop"=w297) -> (w263:T1)
        n74 = Delete From Array(array=w285, index=0 ("Index")) -> (deleted portion=w283:string, array with subset deleted=w282:string[])  [unwired: 1 in]
        n75 = Concatenate Strings(w292, "-pulsedstressV-" ("Substring"), w294, ".txt" ("Substring")) -> (w296:string)
        n76 = VISA Write(VISA resource name=w276, write buffer=":PAGE:CHAN:MODE SWE;" ("write buffer (\"\")"), error in (no error)=w275) -> (VISA resource name out=w273:refnum<visa-resource-name>, error out=w274:errorcluster)  [unwired: 1 out]
        n77 = String To Path(string=w296) -> (path=w291:path)
        n78 = case shown="\"d\", Default" w283 {
          tunnel: [w306 w307] -> w281
          frame "s" {
            w306 = u16 0 items=["Single", "Double"] ("sweep mode")
          }
          frame "d", Default {
            w307 = u16 1 items=["Single", "Double"] ("sweep mode")
          }
        }
        n79 = Fract/Exp String To Number(string=w282) -> (number=w277:dbl[])  [unwired: 3 in, 1 out]
        n80 = Index Array(array=w277, index #1=0 ("Index")) -> (element #1=w253:dbl, element #2=w252:dbl, element #3=w249:dbl, element #4=w248:dbl, element #5=w247:dbl, element #6=w251:dbl)  [unwired: 5 in]
        n81 = Bundle By Name(cluster=w250, "Pulse period"=w248, "Base voltage"=w249, "Pulse width"=w247) -> (w246:T5)
        n82 = Unbundle By Name(w246) -> ("Pulse period"=w254:dbl)
        n83 = Bundle By Name(cluster=w279, "Gate Start"=w252, "Gate Stop"=w253, "Gate Step (linear only)"=0, "Gate Compliance"=w289, "Range mode"=w269, "Range"=w268) -> (w270:T3)
        n84 = call <vilib>:"compatOverwrite.vi"("overwrite (F)"=TRUE) -> ("overwrite?"=w239:T7)
        n85 = Bundle By Name(cluster=w278, "Drain Start"=w251, "Drain Stop"=w244, "Drain Step"=w244, "Drain Compliance"=w290, "Range mode"=w267, "Range"=w266) -> (w271:T4)
        n86 = call <userlib>:"4155C PulsedStressV.vi"("VISA resource name in"=w273, "sweep mode"=w281, "Panel Controls"=w263, "Gate"=w270, "Drain"=w271, "Timings"=w246, "error in (no error)"=w274, "SMU4"=w262) -> ("VISA Resource Name out"=w287:refnum<visa-resource-name>, "ID"=w242:dbl[], "IG"=w240:dbl[], "Outparams"=w264:T8, "error out"=w288:errorcluster)  [unwired: 3 in]
        n87 = Unbundle By Name(w264) -> ("Number of points"=w241:i32)  [unwired: 2 out]
        n88 = for {
          N: w241 -> [_]
          tunnel: [w303] -> w243 mode=indexing
          tunnel: w254 -> [w305]
          i -> [w304]
          n89 = Multiply(x=w305, y=w304) -> (x*y=w303:dbl)
        }
        n90 = Insert Into Array(array=dbl[][] [] ("Input Array"), new element=w243) -> (w255:dbl[][])  [unwired: 2 in]
        n91 = Insert Into Array(array=w255, new element=w242) -> (w260:dbl[][])  [unwired: 2 in]
        n92 = Insert Into Array(array=w260, new element=w240) -> (w259:dbl[][])  [unwired: 2 in]
        n93 = Transpose 2D Array(2D array=w259) -> (transposed array=w258:dbl[][])
        n94 = Open/Create/Replace File(file path (use dialog)=w291, error in=w288, operation (0:open)=w239) -> (refnum out=w300:refnum<file>, error out=w301:errorcluster)  [unwired: 3 in, 1 out]
        n95 = call <userlib>:"4155C Write array to file.vi"("Byte Stream File Refnum"=w300, "Header"=string[] ["Time /s", "Id /A", "Ig /A"], "Data Array"=w258, "error in (no error)"=w301) -> ("dup refnum"=w298:refnum<file>, "error out"=w299:errorcluster)  [unwired: 1 in]
        n96 = Close File(refnum=w298, error in=w299) -> (error out=w286:errorcluster)  [unwired: 1 out]
      }
      frame "transfer-fpp" {
        n97 = Number To Decimal String(number=w362) -> (decimal integer string=w363:string)  [unwired: 1 in]
        n98 = Bundle By Name(cluster=w338, "Emergency Stop"=w367) -> (w375:T6)
        n99 = Delete From Array(array=w353, index=0 ("Index")) -> (deleted portion=w351:string, array with subset deleted=w350:string[])  [unwired: 1 in]
        n100 = Concatenate Strings(w361, "-transferfpp-" ("Substring"), w363, ".txt" ("Substring")) -> (w365:string)
        n101 = VISA Write(VISA resource name=w330, write buffer=":PAGE:CHAN:MODE SWE;" ("write buffer (\"\")"), error in (no error)=w329) -> (VISA resource name out=w327:refnum<visa-resource-name>, error out=w328:errorcluster)  [unwired: 1 out]
        n102 = String To Path(string=w365) -> (path=w360:path)
        n103 = case shown="\"d\", Default" w351 {
          tunnel: [w376 w377] -> w349
          frame "s" {
            w376 = u16 0 items=["Single", "Double"] ("sweep mode")
          }
          frame "d", Default {
            w377 = u16 1 items=["Single", "Double"] ("sweep mode")
          }
        }
        n104 = Fract/Exp String To Number(string=w350) -> (number=w334:dbl[])  [unwired: 3 in, 1 out]
        n105 = Index Array(array=w334, index #1=0 ("Index")) -> (element #1=w348:dbl, element #2=w347:dbl, element #3=w346:dbl)  [unwired: 2 in]
        n106 = Delete From Array(array=w334, length=3 ("Length"), index=0 ("Index")) -> (array with subset deleted=w332:dbl[])  [unwired: 1 out]
        n107 = Bundle By Name(cluster=w340, "Gate Start"=w348, "Gate Stop"=w347, "Gate Step (linear only)"=w346, "Gate Compliance"=w358, "Range mode"=w323, "Range"=w322) -> (w324:T3)
        n108 = Index Array(array=w332, index #1=0 ("Index")) -> (element #1=w343:dbl, element #2=w342:dbl, element #3=w341:dbl)  [unwired: 2 in]
        n109 = call <vilib>:"compatOverwrite.vi"("overwrite (F)"=TRUE) -> ("overwrite?"=w310:T7)
        n110 = Bundle By Name(cluster=w339, "Drain Start"=w343, "Drain Stop"=w342, "Drain Step"=w341, "Drain Compliance"=w359, "Range mode"=w321, "Range"=w320) -> (w325:T4)
        n111 = call <userlib>:"4155C Transfer-FPP.vi"("VISA resource name in"=w327, "Gate"=w324, "Drain"=w325, "Timings"=w357, "error in (no error)"=w328, "sweep mode"=w349, "Panel Controls"=w375) -> ("VG"=w366:dbl[], "Outparams"=w318:T8, "VISA Resource Name out"=w355:refnum<visa-resource-name>, "Vprobe2"=w314:dbl[], "ID"=w313:dbl[], "IG"=w312:dbl[], "Vprobe1"=w311:dbl[], "error out"=w356:errorcluster)  [unwired: 13 in]
        n112 = Unbundle By Name(w318) -> ("V2 Step"=w317:dbl, "V2 Start"=w316:dbl, "Number of points"=w315:i32)
        n113 = Open/Create/Replace File(file path (use dialog)=w360, error in=w356, operation (0:open)=w310) -> (refnum out=w372:refnum<file>, error out=w373:errorcluster)  [unwired: 3 in, 1 out]
        n114 = call <userlib>:"4155C Make Big 2d array FPP.vi"("1D Var1"=w366, "1d ID"=w313, "1d Vp2"=w314, "1d IG"=w312, "1d Vp1"=w311, "VAR2 START"=w316, "Number of VAR2 steps"=w315, "VAR2 STEP"=w317, "VAR1 Name"="Vg", "Decimal places in header"=i8 1, "VAR2 Name"="Vd") -> ("Header array"=w368:string[], "Data array"=w369:dbl[][])  [unwired: 15 in]
        n115 = call <userlib>:"4155C Write array to file.vi"("Byte Stream File Refnum"=w372, "Header"=w368, "Data Array"=w369, "error in (no error)"=w373) -> ("dup refnum"=w370:refnum<file>, "error out"=w371:errorcluster)  [unwired: 1 in]
        n116 = Close File(refnum=w370, error in=w371) -> (error out=w354:errorcluster)  [unwired: 1 out]
      }
      frame "output" {
        n117 = Number To Decimal String(number=w428) -> (decimal integer string=w429:string)  [unwired: 1 in]
        n118 = Bundle By Name(cluster=w404, "Emergency Stop"=w436) -> (w446:T6)
        n119 = Delete From Array(array=w419, index=0 ("Index")) -> (deleted portion=w417:string, array with subset deleted=w416:string[])  [unwired: 1 in]
        n120 = Concatenate Strings(w427, "-output-" ("Substring"), w429, ".txt" ("Substring")) -> (w431:string)
        n121 = VISA Write(VISA resource name=w395, write buffer=":PAGE:CHAN:MODE SWE;" ("write buffer (\"\")"), error in (no error)=w392) -> (VISA resource name out=w394:refnum<visa-resource-name>, error out=w393:errorcluster)  [unwired: 1 out]
        n122 = String To Path(string=w431) -> (path=w426:path)
        n123 = case shown="\"d\", Default" w417 {
          tunnel: [w447 w448] -> w415
          frame "s" {
            w447 = u16 0 items=["Single", "Double"] ("sweep mode")
          }
          frame "d", Default {
            w448 = u16 1 items=["Single", "Double"] ("sweep mode")
          }
        }
        n124 = Fract/Exp String To Number(string=w416) -> (number=w398:dbl[])  [unwired: 3 in, 1 out]
        n125 = Index Array(array=w398, index #1=0 ("Index")) -> (element #1=w414:dbl, element #2=w413:dbl, element #3=w412:dbl)  [unwired: 2 in]
        n126 = Delete From Array(array=w398, length=3 ("Length"), index=0 ("Index")) -> (array with subset deleted=w397:dbl[])  [unwired: 1 out]
        n127 = Bundle By Name(cluster=w406, "Gate Start"=w414, "Gate Stop"=w413, "Gate Step (linear only)"=w412, "Gate Compliance"=w424, "Range mode"=w390, "Range"=w389) -> (w445:T3)
        n128 = Index Array(array=w397, index #1=0 ("Index")) -> (element #1=w409:dbl, element #2=w408:dbl, element #3=w407:dbl)  [unwired: 2 in]
        n129 = call <vilib>:"compatOverwrite.vi"("overwrite (F)"=TRUE) -> ("overwrite?"=w380:T7)
        n130 = Bundle By Name(cluster=w405, "Drain Start"=w409, "Drain Stop"=w408, "Drain Step"=w407, "Drain Compliance"=w425, "Range mode"=w388, "Range"=w391) -> (w444:T4)
        n131 = call <userlib>:"4155C Output.vi"("VISA resource name in"=w394, "Gate"=w445, "Drain"=w444, "Timings"=w423, "error in (no error)"=w393, "SMU4"=w382, "sweep mode"=w415, "Panel controls"=w446) -> ("VD"=w432:dbl[], "Outparams"=w385:T8, "VISA Resource Name out"=w421:refnum<visa-resource-name>, "IS"=w435:dbl[], "ID"=w434:dbl[], "IG"=w433:dbl[], "error out"=w422:errorcluster, "SMU4"=w381:dbl[])  [unwired: 12 in]
        n132 = Unbundle By Name(w385) -> ("V2 Step"=w386:dbl, "V2 Start"=w384:dbl, "Number of points"=w383:i32)
        n133 = Open/Create/Replace File(file path (use dialog)=w426, error in=w422, operation (0:open)=w380) -> (refnum out=w441:refnum<file>, error out=w442:errorcluster)  [unwired: 3 in, 1 out]
        n134 = call <userlib>:"4155C Make Big 2d array.vi"("1D Var1"=w432, "1d IS"=w435, "1d ID"=w434, "1d IG"=w433, "1d SMU4"=w381, "SMU4"=w382, "VAR2 START"=w384, "Number of VAR2 steps"=w383, "VAR2 STEP"=w386, "VAR1 Name"="Vd", "Decimal places in header"=i8 1, "VAR2 Name"="Vg") -> ("Header array"=w437:string[], "Data array"=w438:dbl[][])  [unwired: 14 in]
        n135 = call <userlib>:"4155C Write array to file.vi"("Byte Stream File Refnum"=w441, "Header"=w437, "Data Array"=w438, "error in (no error)"=w442) -> ("dup refnum"=w439:refnum<file>, "error out"=w440:errorcluster)  [unwired: 1 in]
        n136 = Close File(refnum=w439, error in=w440) -> (error out=w420:errorcluster)  [unwired: 1 out]
      }
      frame "output-fpp" {
        n137 = Number To Decimal String(number=w502) -> (decimal integer string=w503:string)  [unwired: 1 in]
        n138 = Bundle By Name(cluster=w478, "Emergency Stop"=w506) -> (w516:T6)
        n139 = Delete From Array(array=w493, index=0 ("Index")) -> (deleted portion=w491:string, array with subset deleted=w490:string[])  [unwired: 1 in]
        n140 = Concatenate Strings(w501, "-outputfpp-" ("Substring"), w503, ".txt" ("Substring")) -> (w505:string)
        n141 = VISA Write(VISA resource name=w469, write buffer=":PAGE:CHAN:MODE SWE;" ("write buffer (\"\")"), error in (no error)=w466) -> (VISA resource name out=w468:refnum<visa-resource-name>, error out=w467:errorcluster)  [unwired: 1 out]
        n142 = String To Path(string=w505) -> (path=w500:path)
        n143 = case shown="\"d\", Default" w491 {
          tunnel: [w517 w518] -> w489
          frame "s" {
            w517 = u16 0 items=["Single", "Double"] ("sweep mode")
          }
          frame "d", Default {
            w518 = u16 1 items=["Single", "Double"] ("sweep mode")
          }
        }
        n144 = Fract/Exp String To Number(string=w490) -> (number=w472:dbl[])  [unwired: 3 in, 1 out]
        n145 = Index Array(array=w472, index #1=0 ("Index")) -> (element #1=w488:dbl, element #2=w487:dbl, element #3=w486:dbl)  [unwired: 2 in]
        n146 = Delete From Array(array=w472, length=3 ("Length"), index=0 ("Index")) -> (array with subset deleted=w471:dbl[])  [unwired: 1 out]
        n147 = Bundle By Name(cluster=w480, "Gate Start"=w488, "Gate Stop"=w487, "Gate Step (linear only)"=w486, "Gate Compliance"=w498, "Range mode"=w464, "Range"=w463) -> (w515:T3)
        n148 = Index Array(array=w471, index #1=0 ("Index")) -> (element #1=w483:dbl, element #2=w482:dbl, element #3=w481:dbl)  [unwired: 2 in]
        n149 = call <vilib>:"compatOverwrite.vi"("overwrite (F)"=TRUE) -> ("overwrite?"=w451:T7)
        n150 = Bundle By Name(cluster=w479, "Drain Start"=w483, "Drain Stop"=w482, "Drain Step"=w481, "Drain Compliance"=w499, "Range mode"=w462, "Range"=w465) -> (w514:T4)
        n151 = call <userlib>:"4155C Output-FPP.vi"("VISA resource name in"=w468, "Gate"=w515, "Drain"=w514, "Timings"=w497, "error in (no error)"=w467, "sweep mode"=w489, "Panel controls"=w516) -> ("VD"=w456:dbl[], "Outparams"=w459:T8, "VISA Resource Name out"=w495:refnum<visa-resource-name>, "Vprobe2"=w455:dbl[], "ID"=w454:dbl[], "IG"=w453:dbl[], "Vprobe1"=w452:dbl[], "error out"=w496:errorcluster)  [unwired: 13 in]
        n152 = Unbundle By Name(w459) -> ("V2 Step"=w460:dbl, "V2 Start"=w458:dbl, "Number of points"=w457:i32)
        n153 = Open/Create/Replace File(file path (use dialog)=w500, error in=w496, operation (0:open)=w451) -> (refnum out=w511:refnum<file>, error out=w512:errorcluster)  [unwired: 3 in, 1 out]
        n154 = call <userlib>:"4155C Make Big 2d array FPP.vi"("1D Var1"=w456, "1d ID"=w454, "1d Vp2"=w455, "1d IG"=w453, "1d Vp1"=w452, "VAR2 START"=w458, "Number of VAR2 steps"=w457, "VAR2 STEP"=w460, "VAR1 Name"="Vd", "Decimal places in header"=i8 1, "VAR2 Name"="Vg") -> ("Header array"=w507:string[], "Data array"=w508:dbl[][])  [unwired: 15 in]
        n155 = call <userlib>:"4155C Write array to file.vi"("Byte Stream File Refnum"=w511, "Header"=w507, "Data Array"=w508, "error in (no error)"=w512) -> ("dup refnum"=w509:refnum<file>, "error out"=w510:errorcluster)  [unwired: 1 in]
        n156 = Close File(refnum=w509, error in=w510) -> (error out=w494:errorcluster)  [unwired: 1 out]
      }
      frame "itime" {
        n157 = Delete From Array(array=w532, index=0 ("Index")) -> (deleted portion=w533:string)  [unwired: 1 in, 1 out]
        n158 = case shown="\"l\"" w533 {
          tunnel: w531 -> [w537 w539 w542]
          tunnel: [w536 w538 w541] -> w524
          frame "s" {
            w535 = u32 0 items=["short  ", "medium  ", "long  "] ("integration time 2")
            n159 = Bundle By Name(cluster=w537, "integration time"=w535) -> (w536:T5)
          }
          frame "m", Default {
            w540 = u32 1 items=["short  ", "medium  ", "long  "] ("integration time 2")
            n160 = Bundle By Name(cluster=w539, "integration time"=w540) -> (w538:T5)
          }
          frame "l" {
            w543 = u32 2 items=["short  ", "medium  ", "long  "] ("integration time 2")
            n161 = Bundle By Name(cluster=w542, "integration time"=w543) -> (w541:T5)
          }
        }
      }
      frame "pulsed" {
        n162 = Delete From Array(array=w558, index=0 ("Index")) -> (deleted portion=w559:string, array with subset deleted=w546:string[])  [unwired: 1 in]
        n163 = case shown="\"on\", Default" w559 {
          tunnel: w557 -> [w569 w572]
          tunnel: [w568 w571] -> w550
          tunnel: w546 -> [w566 _]
          frame "on", Default {
            w567 = u16 1 items=["Continuous", "Pulsed"] ("sweep method")
            n164 = Fract/Exp String To Number(string=w566) -> (number=w564:dbl[])  [unwired: 3 in, 1 out]
            n165 = Index Array(array=w564, index #1=0 ("Index")) -> (element #1=w563:dbl, element #2=w562:dbl, element #3=w561:dbl)  [unwired: 2 in]
            n166 = Bundle By Name(cluster=w569, "sweep method"=w567, "Pulse period"=w563, "Base voltage"=w562, "Pulse width"=w561) -> (w568:T5)
          }
          frame "off" {
            w570 = u16 0 items=["Continuous", "Pulsed"] ("sweep method")
            n167 = Bundle By Name(cluster=w572, "sweep method"=w570) -> (w571:T5)
          }
        }
      }
      frame "gaterangemode" {
        n168 = Delete From Array(array=w585, index=0 ("Index")) -> (deleted portion=w586:string)  [unwired: 1 in, 1 out]
        n169 = case shown="\"f\"" w586 {
          tunnel: [w588 w589 w590] -> w575
          frame "a", Default {
            w588 = u16 0 items=["Auto", "Limited", "Fixed"] ("Gate Range\nmode 2")
          }
          frame "f" {
            w589 = u16 2 items=["Auto", "Limited", "Fixed"] ("Gate Range\nmode 2")
          }
          frame "l" {
            w590 = u16 1 items=["Auto", "Limited", "Fixed"] ("Gate Range\nmode 2")
          }
        }
      }
      frame "gaterange" {
        (unwired) u8 11 items=["10fA  ", "100fA  ", "1nA  ", "10nA", "100nA", "1uA", "10uA", "100uA", "1mA", "10mA", "100mA", "1A"] ("Gate Range 2")
        n170 = Delete From Array(array=w610, index=0 ("Index")) -> (deleted portion=w600:string)  [unwired: 1 in, 1 out]
        n171 = Scan Value(string=w600, format string="") -> (value=w598:dbl)  [unwired: 1 in, 1 out]
        n172 = Logarithm Base 10(1:w598) -> (0:w597:dbl)
        n173 = Round To Nearest(number=w597) -> (nearest integer value=w596:dbl)
        n174 = Add(x=w596, y=11.0) -> (x+y=w594:dbl)
        n175 = To Unsigned Byte Integer(number=w594) -> (unsigned 8bit integer=w593:u8)
      }
      frame "drainrange" {
        (unwired) u8 11 items=["10fA  ", "100fA  ", "1nA  ", "10nA", "100nA", "1uA", "10uA", "100uA", "1mA", "10mA", "100mA", "1A"] ("Gate Range 2")
        n176 = Delete From Array(array=w631, index=0 ("Index")) -> (deleted portion=w622:string)  [unwired: 1 in, 1 out]
        n177 = Scan Value(string=w622, format string="") -> (value=w620:dbl)  [unwired: 1 in, 1 out]
        n178 = Logarithm Base 10(1:w620) -> (0:w619:dbl)
        n179 = Round To Nearest(number=w619) -> (nearest integer value=w618:dbl)
        n180 = Add(x=w618, y=11.0) -> (x+y=w616:dbl)
        n181 = To Unsigned Byte Integer(number=w616) -> (unsigned 8bit integer=w615:u8)
      }
      frame "drainrangemode" {
        n182 = Delete From Array(array=w645, index=0 ("Index")) -> (deleted portion=w646:string)  [unwired: 1 in, 1 out]
        n183 = case shown="\"f\"" w646 {
          tunnel: [w648 w649 w650] -> w635
          frame "a", Default {
            w648 = u16 0 items=["Auto", "Limited", "Fixed"] ("Gate Range\nmode 2")
          }
          frame "f" {
            w649 = u16 2 items=["Auto", "Limited", "Fixed"] ("Gate Range\nmode 2")
          }
          frame "l" {
            w650 = u16 1 items=["Auto", "Limited", "Fixed"] ("Gate Range\nmode 2")
          }
        }
      }
      frame "Error", Default {
      }
      frame "logfile" {
        n184 = Number To Decimal String(number=w695) -> (decimal integer string=w699:string)  [unwired: 1 in]
        n185 = Concatenate Strings(w697, "logfile" ("Substring"), w699, ".txt" ("Substring")) -> (w694:string)
        n186 = String To Path(string=w694) -> (path=w667:path)
        n187 = Unbundle(w693) -> ("integration time"=w692:u32, "Short/Long integration time"=w691:dbl, "hold time (sec)"=w690:dbl, "delay time (sec)"=w689:dbl, "Step Time (0 disables)"=w688:dbl, "sweep method"=w687:u16, "Pulse period"=w686:dbl, "Base voltage"=w685:dbl, "Pulse width"=w684:dbl)
        n188 = Build Array(w692, w691, w690, w689, w688, w687, w686, w685, w684, w678, w679, w680, w681, w682, w683) -> (w671:dbl[])
        n189 = Insert Into Array(array=dbl[][] [] ("Input Array"), new element=w671) -> (w670:dbl[][])  [unwired: 2 in]
        n190 = call <vilib>:"compatOverwrite.vi"("overwrite (F)"=TRUE) -> ("overwrite?"=w665:T7)
        n191 = Open/Create/Replace File(file path (use dialog)=w667, error in=w669, operation (0:open)=w665) -> (refnum out=w675:refnum<file>, error out=w674:errorcluster)  [unwired: 3 in, 1 out]
        n192 = call <userlib>:"4155C Write array to file.vi"("Byte Stream File Refnum"=w675, "Header"=string[] ["Int Time", "Short/Long Itime", "Hold time", "Delay time", "Step time", "Sweep method", "Pulse period", "Base Voltage", "Pulse width", "Drain compliance", "Gate compliance", "Gate range mode", "Gate range", "S/D range mode", "S/D range"], "Data Array"=w670, "error in (no error)"=w674) -> ("dup refnum"=w677:refnum<file>, "error out"=w676:errorcluster)  [unwired: 1 in]
        n193 = Close File(refnum=w677, error in=w676) -> (error out=w668:errorcluster)  [unwired: 1 out]
      }
      frame "sample" {
        n194 = Number To Decimal String(number=w750) -> (decimal integer string=w749:string)  [unwired: 1 in]
        n195 = Fract/Exp String To Number(string=w746) -> (number=w706:dbl[])  [unwired: 3 in, 1 out]
        n196 = Concatenate Strings(w724, "-sample-" ("Substring"), w749, ".txt" ("Substring")) -> (w747:string)
        n197 = String To Path(string=w747) -> (path=w728:path)
        n198 = Index Array(array=w706, index=0 ("Index")) -> (element=w744:dbl)
        n199 = Index Array(array=w706, index=2 ("Index")) -> (element=w740:dbl)
        n200 = Index Array(array=w706, index=3 ("Index")) -> (element=w709:dbl)
        n201 = Index Array(array=w706, index=4 ("Index")) -> (element=w705:dbl)
        n202 = call <userlib>:"4155C Config Sampling Measurements.vi"("Sampling interval"=w705, "Sample time"=w709, "Display on/off"=TRUE, "Timings"=w715, "Num Points"=w740, "error in (no error)"=w752, "Drain Compliance"=w751, "Gate Compliance"=w725, "VISA session"=w753) -> ("error out"=w754:errorcluster, "dup VISA resource name"=w755:refnum<visa-resource-name>)  [unwired: 1 in]
        n203 = Index Array(array=w706, index=1 ("Index")) -> (element=w741:dbl)
        n204 = call <userlib>:"4155C Take Sample.vi"("Emergency Stop"=w721, "error in (no error)"=w754, "Vd"=w741, "Vg"=w744, "VISA resource name in"=w755) -> ("error out"=w719:errorcluster, "Id"=w757:dbl[], "Ig"=w730:dbl[], "VISA Resource Name out"=w717:refnum<visa-resource-name>, "Is"=w756:dbl[], "Time"=w734:dbl[])  [unwired: 1 in]
        n205 = Insert Into Array(array=dbl[][] [] ("Input Array"), new element=w734) -> (w733:dbl[][])  [unwired: 2 in]
        n206 = Insert Into Array(array=w733, new element=w730) -> (w732:dbl[][])  [unwired: 2 in]
        n207 = Insert Into Array(array=w732, new element=w757) -> (w731:dbl[][])  [unwired: 2 in]
        n208 = VISA Write(VISA resource name=w717, write buffer=":DISP ON" ("write buffer (\"\")"), error in (no error)=w719) -> (VISA resource name out=w716:refnum<visa-resource-name>, error out=w718:errorcluster)  [unwired: 1 out]
        n209 = Insert Into Array(array=w731, new element=w756) -> (w723:dbl[][])  [unwired: 2 in]
        n210 = Transpose 2D Array(2D array=w723) -> (transposed array=w722:dbl[][])
        n211 = call <vilib>:"compatOverwrite.vi"("overwrite (F)"=TRUE) -> ("overwrite?"=w703:T7)
        n212 = Open/Create/Replace File(file path (use dialog)=w728, error in=w718, operation (0:open)=w703) -> (refnum out=w737:refnum<file>, error out=w736:errorcluster)  [unwired: 3 in, 1 out]
        n213 = call <userlib>:"4155C Write array to file.vi"("Byte Stream File Refnum"=w737, "Header"=string[] ["Time /s", "Ig /A", "Id /A", "Is /A"], "Data Array"=w722, "error in (no error)"=w736) -> ("dup refnum"=w739:refnum<file>, "error out"=w738:errorcluster)  [unwired: 1 in]
        n214 = Close File(refnum=w739, error in=w738) -> (error out=w726:errorcluster)  [unwired: 1 out]
      }
      frame "samplei" {
        n215 = Number To Decimal String(number=w810) -> (decimal integer string=w809:string)  [unwired: 1 in]
        n216 = Fract/Exp String To Number(string=w806) -> (number=w772:dbl[])  [unwired: 3 in, 1 out]
        n217 = Concatenate Strings(w788, "-samplei-" ("Substring"), w809, ".txt" ("Substring")) -> (w807:string)
        n218 = String To Path(string=w807) -> (path=w791:path)
        n219 = Index Array(array=w772, index=4 ("Index")) -> (element=w766:dbl)
        n220 = Index Array(array=w772, index=3 ("Index")) -> (element=w767:dbl)
        n221 = Index Array(array=w772, index=1 ("Index")) -> (element=w769:dbl)
        n222 = Index Array(array=w772, index=0 ("Index")) -> (element=w770:dbl)
        n223 = Index Array(array=w772, index=2 ("Index")) -> (element=w768:dbl)
        n224 = call <userlib>:"4155C Config SamplingI Measurements.vi"("Sample time"=w768, "Display on/off"=TRUE, "Timings"=w780, "Num Points"=w769, "error in (no error)"=w812, "Sampling interval"=w767, "VISA session"=w813) -> ("error out"=w814:errorcluster, "dup VISA resource name"=w815:refnum<visa-resource-name>)  [unwired: 3 in]
        n225 = call <userlib>:"4155C Take SampleI.vi"("Emergency Stop"=w785, "error in (no error)"=w814, "Idg 2"=w770, "Vdg compliance 2"=w766, "VISA resource name in"=w815) -> ("error out"=w783:errorcluster, "Idg"=w817:dbl[], "Vdg"=w793:dbl[], "VISA Resource Name out"=w781:refnum<visa-resource-name>, "Is"=w816:dbl[], "Time"=w797:dbl[])  [unwired: 1 in]
        n226 = Insert Into Array(array=dbl[][] [] ("Input Array"), new element=w797) -> (w796:dbl[][])  [unwired: 2 in]
        n227 = Insert Into Array(array=w796, new element=w793) -> (w795:dbl[][])  [unwired: 2 in]
        n228 = Insert Into Array(array=w795, new element=w817) -> (w794:dbl[][])  [unwired: 2 in]
        n229 = VISA Write(VISA resource name=w781, write buffer=":DISP ON" ("write buffer (\"\")"), error in (no error)=w783) -> (VISA resource name out=w765:refnum<visa-resource-name>, error out=w782:errorcluster)  [unwired: 1 out]
        n230 = Insert Into Array(array=w794, new element=w816) -> (w787:dbl[][])  [unwired: 2 in]
        n231 = Transpose 2D Array(2D array=w787) -> (transposed array=w786:dbl[][])
        n232 = call <vilib>:"compatOverwrite.vi"("overwrite (F)"=TRUE) -> ("overwrite?"=w760:T7)
        n233 = Open/Create/Replace File(file path (use dialog)=w791, error in=w782, operation (0:open)=w760) -> (refnum out=w800:refnum<file>, error out=w799:errorcluster)  [unwired: 3 in, 1 out]
        n234 = call <userlib>:"4155C Write array to file.vi"("Byte Stream File Refnum"=w800, "Header"=string[] ["Time /s", "Vdg /V", "Idg /A", "Is /A"], "Data Array"=w786, "error in (no error)"=w799) -> ("dup refnum"=w802:refnum<file>, "error out"=w801:errorcluster)  [unwired: 1 in]
        n235 = Close File(refnum=w802, error in=w801) -> (error out=w763:errorcluster)  [unwired: 1 out]
        n236 = VISA Write(VISA resource name=w765, write buffer=";:PAGE:SCON:STAN OFF;:PAGE:CHAN:VSU2:DIS;" ("write buffer (\"\")"), error in (no error)=w763) -> (VISA resource name out=w761:refnum<visa-resource-name>, error out=w762:errorcluster)  [unwired: 1 out]
      }
      frame "#" {
        n237 = VISA Write(VISA resource name=w824, write buffer=":DISP ON" ("write buffer (\"\")"), error in (no error)=w823) -> (VISA resource name out=w822:refnum<visa-resource-name>, error out=w821:errorcluster)  [unwired: 1 out]
      }
      frame "stressV" {
        n238 = Number To Decimal String(number=w874) -> (decimal integer string=w873:string)  [unwired: 1 in]
        n239 = Fract/Exp String To Number(string=w870) -> (number=w842:dbl[])  [unwired: 3 in, 1 out]
        n240 = Concatenate Strings(w857, "-stressV-" ("Substring"), w873, ".txt" ("Substring")) -> (w871:string)
        n241 = String To Path(string=w871) -> (path=w861:path)
        n242 = Index Array(array=w842, index=3 ("Index")) -> (element=w839:dbl)
        n243 = Index Array(array=w842, index=1 ("Index")) -> (element=w837:dbl)
        n244 = Index Array(array=w842, index=0 ("Index")) -> (element=w836:dbl)
        n245 = Index Array(array=w842, index=4 ("Index")) -> (element=w841:dbl)
        n246 = Index Array(array=w842, index=2 ("Index")) -> (element=w838:dbl)
        n247 = call <userlib>:"4155C Config V Stress.vi"("VISA session"=w877, "ID compliance"=w839, "VD"=w837, "VG"=w836, "IG compliance"=w838, "error in (no error)"=w876, "Display on/off"=TRUE) -> ("dup VISA resource name"=w879:refnum<visa-resource-name>, "error out"=w878:errorcluster)
        n248 = call <userlib>:"4155C Apply Stress.vi"("error in (no error)"=w878, "Duration"=w841, "Emergency Stop"=w856, "VISA resource name in"=w879) -> ("error out"=w854:errorcluster, "VISA Resource Name out"=w852:refnum<visa-resource-name>)
        n249 = VISA Write(VISA resource name=w852, write buffer=":DISP ON" ("write buffer (\"\")"), error in (no error)=w854) -> (VISA resource name out=w851:refnum<visa-resource-name>, error out=w853:errorcluster)  [unwired: 1 out]
        n250 = call <vilib>:"compatOverwrite.vi"("overwrite (F)"=TRUE) -> ("overwrite?"=w835:T7)
        n251 = Open/Create/Replace File(file path (use dialog)=w861, error in=w853, operation (0:open)=w835) -> (refnum out=w864:refnum<file>, error out=w863:errorcluster)  [unwired: 3 in, 1 out]
        n252 = call <userlib>:"4155C Write array to file.vi"("Byte Stream File Refnum"=w864, "Header"=string[] ["V stress completed successfully", ""], "error in (no error)"=w863) -> ("dup refnum"=w866:refnum<file>, "error out"=w865:errorcluster)  [unwired: 2 in]
        n253 = Close File(refnum=w866, error in=w865) -> (error out=w859:errorcluster)  [unwired: 1 out]
      }
      frame "stressI" {
        n254 = Number To Decimal String(number=w917) -> (decimal integer string=w916:string)  [unwired: 1 in]
        n255 = Fract/Exp String To Number(string=w913) -> (number=w887:dbl[])  [unwired: 3 in, 1 out]
        n256 = Concatenate Strings(w900, "-stressI-" ("Substring"), w916, ".txt" ("Substring")) -> (w914:string)
        n257 = String To Path(string=w914) -> (path=w904:path)
        n258 = Index Array(array=w887, index=1 ("Index")) -> (element=w883:dbl)
        n259 = Index Array(array=w887, index=0 ("Index")) -> (element=w884:dbl)
        n260 = call <userlib>:"4155C Config I Stress.vi"("VISA session"=w920, "IDG"=w884, "VDG compliance"=w883, "error in (no error)"=w919, "Display on/off"=TRUE) -> ("dup VISA resource name"=w922:refnum<visa-resource-name>, "error out"=w921:errorcluster)
        n261 = Index Array(array=w887, index=2 ("Index")) -> (element=w885:dbl)
        n262 = call <userlib>:"4155C Apply Stress.vi"("error in (no error)"=w921, "Duration"=w885, "Emergency Stop"=w899, "VISA resource name in"=w922) -> ("error out"=w897:errorcluster, "VISA Resource Name out"=w895:refnum<visa-resource-name>)
        n263 = VISA Write(VISA resource name=w895, write buffer=":DISP ON" ("write buffer (\"\")"), error in (no error)=w897) -> (VISA resource name out=w894:refnum<visa-resource-name>, error out=w896:errorcluster)  [unwired: 1 out]
        n264 = call <vilib>:"compatOverwrite.vi"("overwrite (F)"=TRUE) -> ("overwrite?"=w882:T7)
        n265 = Open/Create/Replace File(file path (use dialog)=w904, error in=w896, operation (0:open)=w882) -> (refnum out=w907:refnum<file>, error out=w906:errorcluster)  [unwired: 3 in, 1 out]
        n266 = call <userlib>:"4155C Write array to file.vi"("Byte Stream File Refnum"=w907, "Header"=string[] ["I stress completed successfully", ""], "error in (no error)"=w906) -> ("dup refnum"=w909:refnum<file>, "error out"=w908:errorcluster)  [unwired: 2 in]
        n267 = Close File(refnum=w909, error in=w908) -> (error out=w902:errorcluster)  [unwired: 1 out]
      }
      frame "vsu2pulse" {
        n268 = Number To Decimal String(number=w958) -> (decimal integer string=w957:string)  [unwired: 1 in]
        n269 = Fract/Exp String To Number(string=w954) -> (number=w929:dbl[])  [unwired: 3 in, 1 out]
        n270 = Concatenate Strings(w942, "-vsu2-" ("Substring"), w957, ".txt" ("Substring")) -> (w955:string)
        n271 = String To Path(string=w955) -> (path=w946:path)
        n272 = Index Array(array=w929, index=1 ("Index")) -> (element=w928:dbl)
        n273 = Index Array(array=w929, index=0 ("Index")) -> (element=w926:dbl)
        n274 = call <userlib>:"4155C Config VSU2 Stress.vi"("error in (no error)"=w960, "VSU2"=w926, "Display on/off"=TRUE, "VISA session"=w961) -> ("error out"=w962:errorcluster, "dup VISA resource name"=w963:refnum<visa-resource-name>)
        n275 = call <userlib>:"4155C Apply Stress.vi"("error in (no error)"=w962, "Duration"=w928, "Emergency Stop"=w941, "VISA resource name in"=w963) -> ("error out"=w939:errorcluster, "VISA Resource Name out"=w937:refnum<visa-resource-name>)
        n276 = VISA Write(VISA resource name=w937, write buffer=":DISP ON" ("write buffer (\"\")"), error in (no error)=w939) -> (VISA resource name out=w936:refnum<visa-resource-name>, error out=w938:errorcluster)  [unwired: 1 out]
        n277 = call <vilib>:"compatOverwrite.vi"("overwrite (F)"=TRUE) -> ("overwrite?"=w925:T7)
        n278 = Open/Create/Replace File(file path (use dialog)=w946, error in=w938, operation (0:open)=w925) -> (refnum out=w949:refnum<file>, error out=w948:errorcluster)  [unwired: 3 in, 1 out]
        n279 = call <userlib>:"4155C Write array to file.vi"("Byte Stream File Refnum"=w949, "Header"=string[] ["VSU2 pulse completed successfully", ""], "error in (no error)"=w948) -> ("dup refnum"=w951:refnum<file>, "error out"=w950:errorcluster)  [unwired: 2 in]
        n280 = Close File(refnum=w951, error in=w950) -> (error out=w944:errorcluster)  [unwired: 1 out]
      }
      frame "sample-fpp" {
        w973 = string[] ["Time /s", "Id VgVd /A", "Ig VgVd /A", "Vp1 VgVd /V", "Vp2 VgVd /V"] ("Header")
        w977 = "%d" ("format string")
        n281 = Number To Decimal String(number=w1027) -> (decimal integer string=w1026:string)  [unwired: 1 in]
        n282 = Fract/Exp String To Number(string=w1023) -> (number=w1011:dbl[])  [unwired: 3 in, 1 out]
        n283 = Concatenate Strings(w1017, "-samplefpp-" ("Substring"), w1026, ".txt" ("Substring")) -> (w1024:string)
        n284 = String To Path(string=w1024) -> (path=w985:path)
        n285 = Index Array(array=w1011, index=0 ("Index")) -> (element=w971:dbl)
        n286 = Index Array(array=w1011, index=1 ("Index")) -> (element=w970:dbl)
        n287 = Index Array(array=w1011, index=2 ("Index")) -> (element=w1019:dbl)
        n288 = Index Array(array=w1011, index=3 ("Index")) -> (element=w1009:dbl)
        n289 = call <userlib>:"4155C Config Sampling Measurements FPP.vi"("VISA session"=w1030, "Num Points"=w1019, "Vg"=w971, "Display on/off"=TRUE, "Gate Compliance"=w1018, "Drain Compliance"=w1028, "Standby"="Standby", "error in (no error)"=w1029, "Timings"=w1016, "Vd"=w970, "Sample time"=w1009) -> ("dup VISA resource name"=w987:refnum<visa-resource-name>, "error out"=w986:errorcluster)  [unwired: 3 in]
        n290 = Number To Decimal String(number=w971) -> (decimal integer string=w997:string)  [unwired: 1 in]
        n291 = call <userlib>:"4155C Take Sample FPP.vi"("VISA resource name in"=w987, "error in (no error)"=w986, "Emergency Stop"=w988) -> ("Time"=w992:dbl[], "Vp1"=w1002:dbl[], "VISA Resource Name out"=w968:refnum<visa-resource-name>, "Ig"=w990:dbl[], "Id"=w991:dbl[], "Vp2"=w1000:dbl[], "error out"=w989:errorcluster)  [unwired: 10 in]
        n292 = Insert Into Array(array=dbl[][] [] ("Input Array"), new element=w992) -> (w1006:dbl[][])  [unwired: 2 in]
        n293 = Number To Decimal String(number=w970) -> (decimal integer string=w995:string)  [unwired: 1 in]
        n294 = Insert Into Array(array=w1006, new element=w991) -> (w1005:dbl[][])  [unwired: 2 in]
        n295 = Concatenate Strings("(Vg = " ("Substring"), w997, "V, Vd = " ("Substring"), w995, "V)" ("Substring")) -> (w993:string)
        n296 = Insert Into Array(array=w1005, new element=w990) -> (w1004:dbl[][])  [unwired: 2 in]
        n297 = Insert Into Array(array=w1004, new element=w1002) -> (w1001:dbl[][])  [unwired: 2 in]
        n298 = Insert Into Array(array=w1001, new element=w1000) -> (w969:dbl[][])  [unwired: 2 in]
        n299 = call <vilib>:"compatOverwrite.vi"("overwrite (F)"=TRUE) -> ("overwrite?"=w966:T7)
        n300 = Open/Create/Replace File(file path (use dialog)=w985, error in=w989, operation (0:open)=w966) -> (refnum out=w982:refnum<file>, error out=w983:errorcluster)  [unwired: 3 in, 1 out]
        n301 = Array To Spreadsheet String(array=w973, 3:w977) -> (spreadsheet string=w979:string)  [unwired: 1 in]
        n302 = Transpose 2D Array(2D array=w969) -> (transposed array=w999:dbl[][])
        n303 = Search and Replace String(replace all?=TRUE ("replace all? (F)"), input string=w979, search string="VgVd", replace string=w993) -> (result string=w975:string)  [unwired: 4 in, 3 out]
        n304 = Spreadsheet String To Array(format string=w977, spreadsheet string=w975, array type (2D Dbl)=w973) -> (array=w974:string[])  [unwired: 1 in]
        n305 = call <userlib>:"4155C Write array to file.vi"("Byte Stream File Refnum"=w982, "Header"=w974, "Data Array"=w999, "error in (no error)"=w983) -> ("dup refnum"=w980:refnum<file>, "error out"=w981:errorcluster)  [unwired: 1 in]
        n306 = Close File(refnum=w980, error in=w981) -> (error out=w967:errorcluster)  [unwired: 1 out]
      }
      frame "resample-fpp" {
        w1042 = string[] ["Time /s", "Id VgVd /A", "Ig VgVd /A", "Vp1 VgVd /V", "Vp2 VgVd /V"] ("Header")
        w1046 = "%d" ("format string")
        n307 = Number To Decimal String(number=w1088) -> (decimal integer string=w1087:string)  [unwired: 1 in]
        n308 = Fract/Exp String To Number(string=w1084) -> (number=w1035:dbl[])  [unwired: 3 in, 1 out]
        n309 = Concatenate Strings(w1080, "-resamplefpp-" ("Substring"), w1087, ".txt" ("Substring")) -> (w1085:string)
        n310 = String To Path(string=w1085) -> (path=w1054:path)
        n311 = Index Array(array=w1035, index=0 ("Index")) -> (element=w1041:dbl)
        n312 = Index Array(array=w1035, index=1 ("Index")) -> (element=w1040:dbl)
        n313 = Number To Decimal String(number=w1041) -> (decimal integer string=w1064:string)  [unwired: 1 in]
        n314 = call <userlib>:"4155C Take Sample FPP.vi"("VISA resource name in"=w1037, "error in (no error)"=w1036, "Emergency Stop"=w1055) -> ("Time"=w1059:dbl[], "Vp1"=w1069:dbl[], "VISA Resource Name out"=w1039:refnum<visa-resource-name>, "Ig"=w1057:dbl[], "Id"=w1058:dbl[], "Vp2"=w1067:dbl[], "error out"=w1056:errorcluster)  [unwired: 10 in]
        n315 = Insert Into Array(array=dbl[][] [] ("Input Array"), new element=w1059) -> (w1073:dbl[][])  [unwired: 2 in]
        n316 = Number To Decimal String(number=w1040) -> (decimal integer string=w1062:string)  [unwired: 1 in]
        n317 = Insert Into Array(array=w1073, new element=w1058) -> (w1072:dbl[][])  [unwired: 2 in]
        n318 = Concatenate Strings("(Vg = " ("Substring"), w1064, "V, Vd = " ("Substring"), w1062, "V)" ("Substring")) -> (w1060:string)
        n319 = Insert Into Array(array=w1072, new element=w1057) -> (w1071:dbl[][])  [unwired: 2 in]
        n320 = Insert Into Array(array=w1071, new element=w1069) -> (w1068:dbl[][])  [unwired: 2 in]
        n321 = Insert Into Array(array=w1068, new element=w1067) -> (w1034:dbl[][])  [unwired: 2 in]
        n322 = call <vilib>:"compatOverwrite.vi"("overwrite (F)"=TRUE) -> ("overwrite?"=w1033:T7)
        n323 = Open/Create/Replace File(file path (use dialog)=w1054, error in=w1056, operation (0:open)=w1033) -> (refnum out=w1051:refnum<file>, error out=w1052:errorcluster)  [unwired: 3 in, 1 out]
        n324 = Array To Spreadsheet String(array=w1042, 3:w1046) -> (spreadsheet string=w1048:string)  [unwired: 1 in]
        n325 = Transpose 2D Array(2D array=w1034) -> (transposed array=w1066:dbl[][])
        n326 = Search and Replace String(replace all?=TRUE ("replace all? (F)"), input string=w1048, search string="VgVd", replace string=w1060) -> (result string=w1044:string)  [unwired: 4 in, 3 out]
        n327 = Spreadsheet String To Array(format string=w1046, spreadsheet string=w1044, array type (2D Dbl)=w1042) -> (array=w1043:string[])  [unwired: 1 in]
        n328 = call <userlib>:"4155C Write array to file.vi"("Byte Stream File Refnum"=w1051, "Header"=w1043, "Data Array"=w1066, "error in (no error)"=w1052) -> ("dup refnum"=w1049:refnum<file>, "error out"=w1050:errorcluster)  [unwired: 1 in]
        n329 = Close File(refnum=w1049, error in=w1050) -> (error out=w1038:errorcluster)  [unwired: 1 out]
      }
    }
  }
  "error out" <- w1
